vi "SetId.vi"(8 "error in (no error)":errorcluster, 10 "Id":string, 11 "LinkingHeadingId in":refnum<class "LinkingHeadingId.lvclass">) -> (0 "error out":errorcluster, 3 "LinkingHeadingId out":refnum<class "LinkingHeadingId.lvclass">)   [LabVIEW 2021, in "LvMarkdown.lvlib" / "LinkingHeadingId.lvclass"]
uses:
  LinkingHeadingId.lvclass
  LinkingHeadingId.lvclass/LinkingHeadingId.ctl
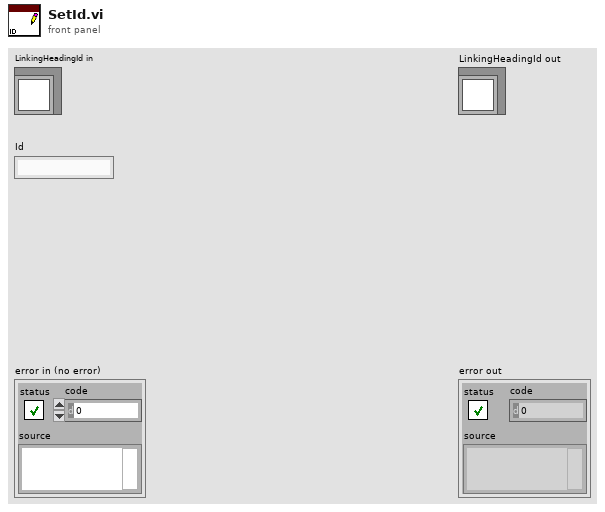
[diagram p1: front panel]
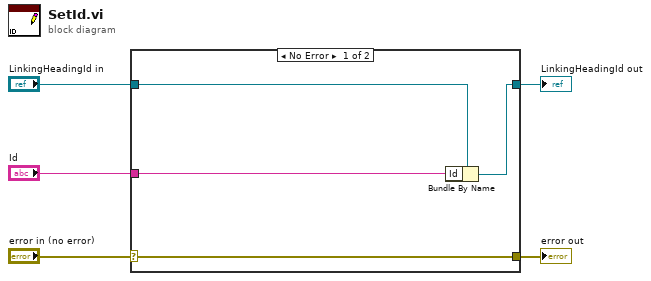
[diagram p0: block diagram]
diagram:
  n1 = case shown="No Error" "error in (no error)" {
    selector: "error in (no error)" -> [w9 w10]
    tunnel: [w9 w10] -> w4
    tunnel: [w7 w11] -> w2
    tunnel: "LinkingHeadingId in" -> [w8 w11]
    tunnel: "Id" -> [w6 _]
    frame No Error {
      n2 = Bundle By Name(cluster=w8, "Id"=w6) -> (w7:refnum<class "LinkingHeadingId.lvclass">)
    }
    frame Error {
    }
  }
  "error out" <- w4
  "LinkingHeadingId out" <- w2
